vi "Actor Core.vi"(8 "error in":errorcluster, 11 "Measure Object in":refnum<class "TDMS Properties.lvclass">) -> (0 "error out":errorcluster, 3 "Actor out":refnum<class "Actor.lvclass">)   [LabVIEW 2019, in "TDMS Properties.lvclass"]
doc: "(<B>Filename</B>: Actor Framework.lvlib:Actor.lvclass:Actor Core.vi)\n\nReceives messages to the actor, reacts to them, and initiates any error handling that may shut the actor down.\n\nDescendant classes may override this VI to append parallel tasks for the actor to complete while it handles messages. Overrides use the Call Parent Method node."
uses:
  TDMS Properties.lvclass
  C:/GitHub/LabActor/Template Module/Template Module.lvclass
  C:/Program Files/National Instruments/LabVIEW 2019/vi.lib/ActorFramework/Actor/Actor.lvclass
  <vilib>/ActorFramework/Actor/Actor.lvclass
  <vilib>/Utility/tdmsutil.llb/fileViewerConfigData.ctl
  TDMS Properties.lvclass/TDMS Properties.ctl
  Template Module/Template Module.lvclass/Template Module.ctl
  <vilib>/ActorFramework/Actor/Actor.lvclass/Actor.ctl
  <vilib>/ActorFramework/Message Enqueuer/Message Enqueuer.lvclass/Message Enqueuer.ctl
  <vilib>/Utility/error.llb/DialogType.ctl
  Read File.vi
  Template Module/Read stop event.vi
  <vilib>/ActorFramework/Message Enqueuer/Init from Existing Queue.vi
  <vilib>/ActorFramework/Message Enqueuer/Enqueue.vi
  <vilib>/ActorFramework/Stop Msg/Stop Msg.lvclass
  C:/Program Files/National Instruments/LabVIEW 2019/vi.lib/ActorFramework/Message/Message.lvclass
  <vilib>/ActorFramework/Message Priority Queue/Priority Enqueue.vi
  Template Module/Template Module.lvclass
  <vilib>/ActorFramework/Message Enqueuer/Message Enqueuer.lvclass
panel:
  in  "Quit":bool
  in  "Properties":i32(listbox)
  out "file path out":path
  in  "File contents":string(tree)
  in  "Settings...":bool
  in  "Status":string
  in  "Help":bool
  in  "LastTopLeftValue":u64
  out "Temp Configuration":T1
  out "TotalCount":u64
  out "LastXScaleFormat":u8
  in  "Properties / Values / Graph":T2(tab)
  in  "Go To":bool
  in  "Scrollbar":u64(c297)
  in  "Raw data values":i32(listbox)
  out "Waveform Graph":waveform(dbl)[](graph)
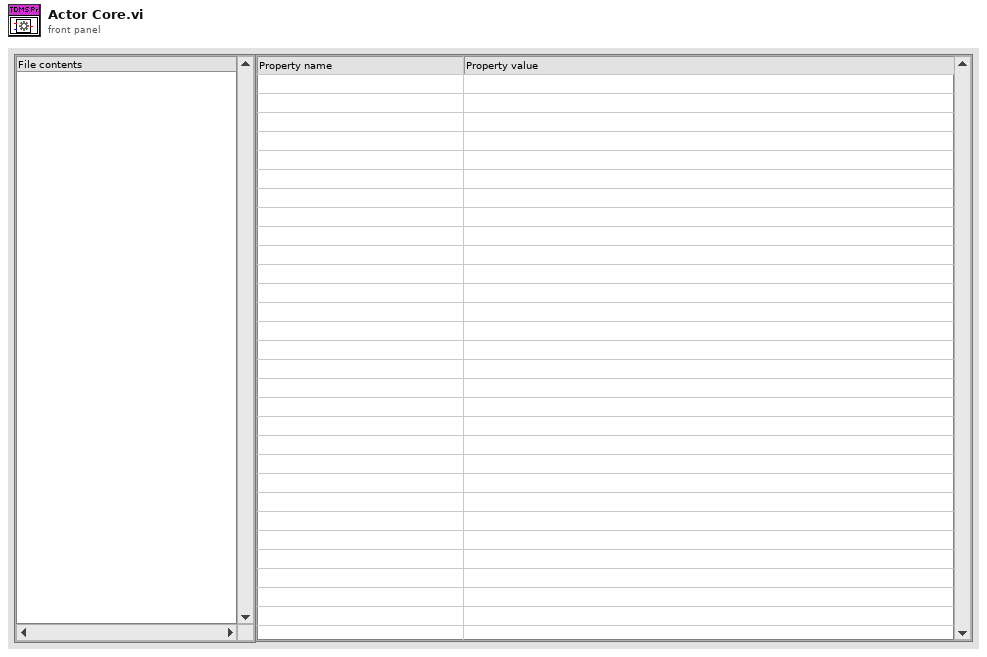
[diagram p1: front panel]
types:
  T1 = typedef "fileViewerConfigData.ctl" = cluster{"Show all (table)":bool, "Show all (graph)":bool, "limit (table)":u64, "limit (graph)":u64, "no show":bool, "start (table)":u64, "start (graph)":u64}
  T2 = enum32{"Properties", "Values (table)", "Analog values (graph)"}
  T3 = enum16{"open", "open or create", "create or replace", "create", "open (read-only)"}
  T4 = cluster{"Tree":refnum<vi>, "Tab Control":refnum<vi>, "property list":refnum<vi>, "raw data list":refnum<vi>, "Waveform Graph":refnum<vi>, "Ok":refnum<vi>, "Ok 2":refnum<vi>, "Ok 3":refnum<vi>, "Ok 4":refnum<vi>, "Scrollbar":refnum<vi>, "Ok 5":refnum<vi>, "TopLeftValue":refnum<vi>, "TotalCount":refnum<vi>}
  T5 = typedef "DialogType.ctl" = u16
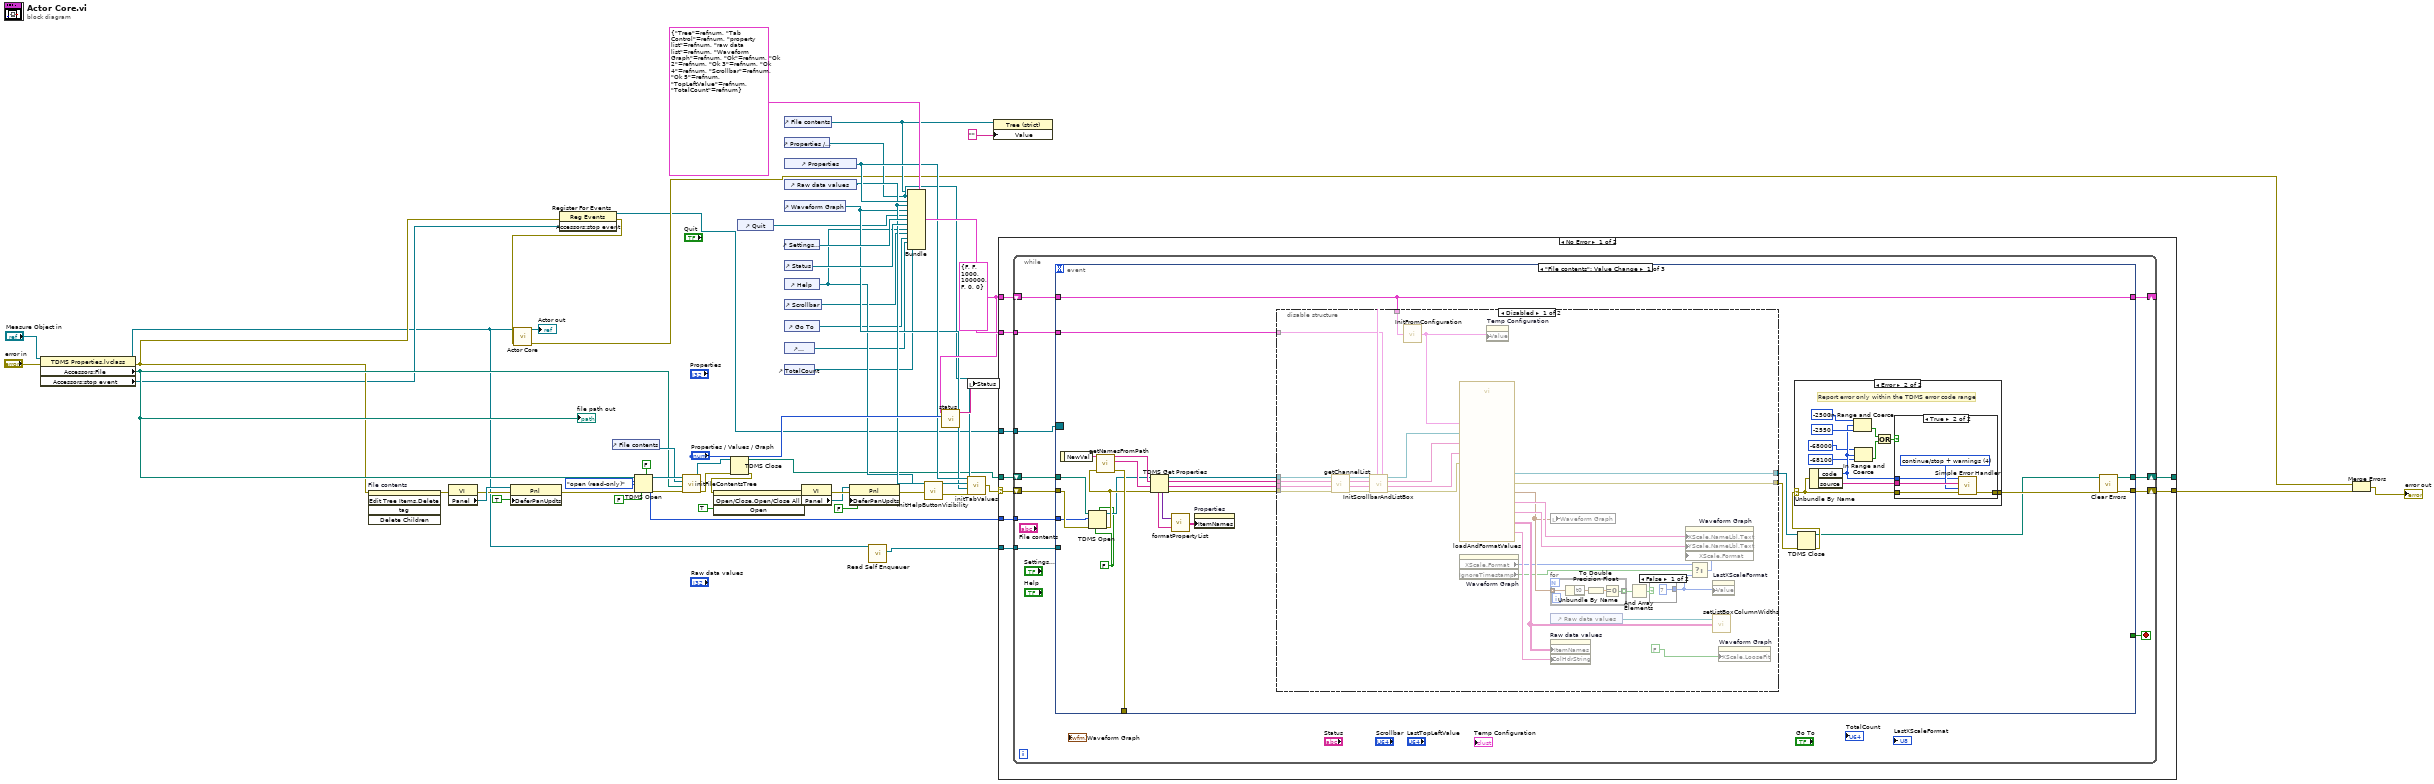
[diagram p0: block diagram]
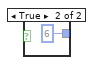
[diagram p2: hidden frame]
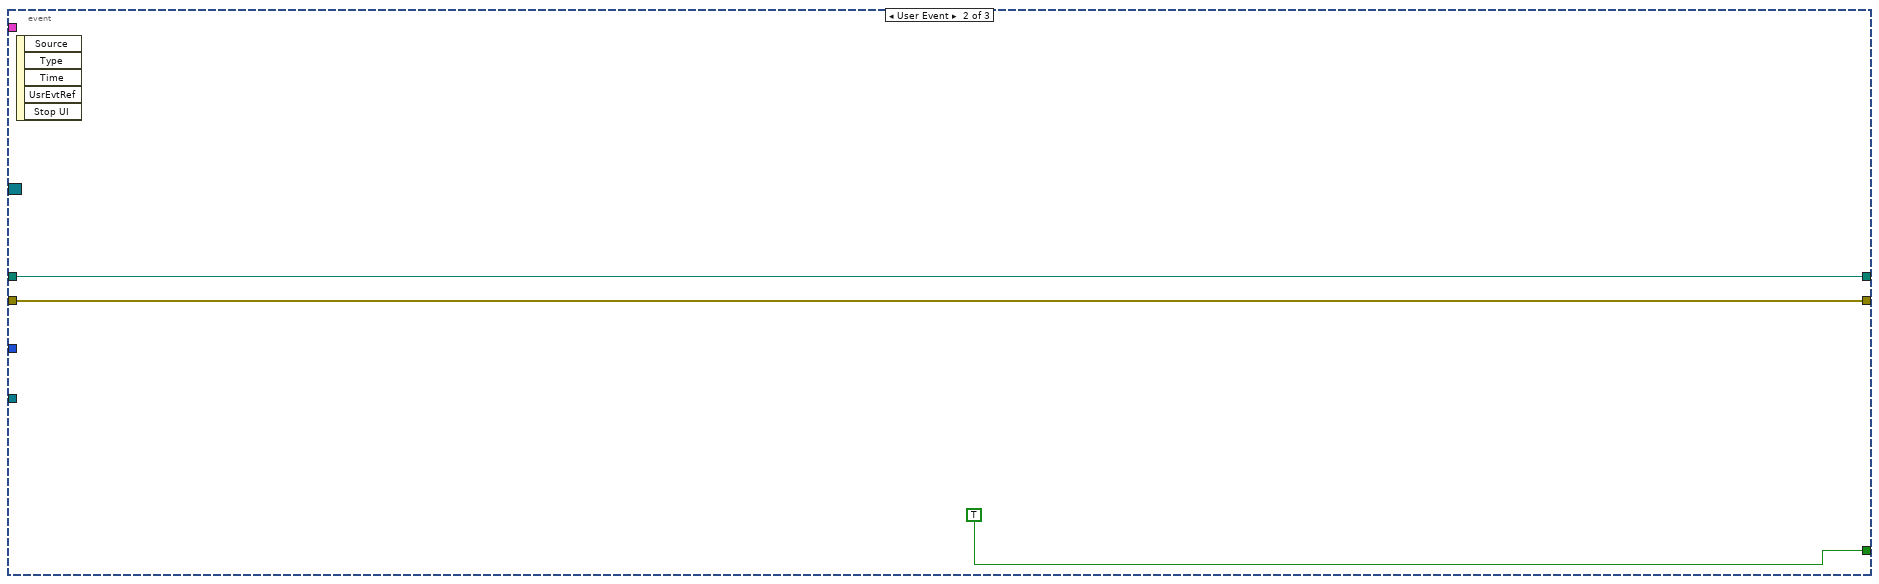
[diagram p6: hidden frame]
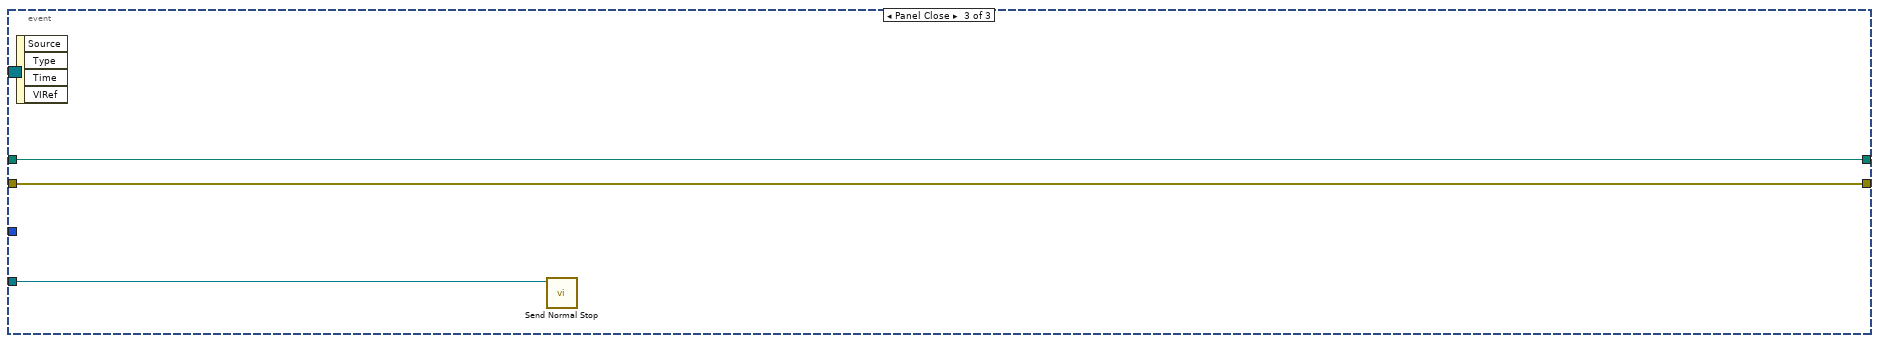
[diagram p7: hidden frame]
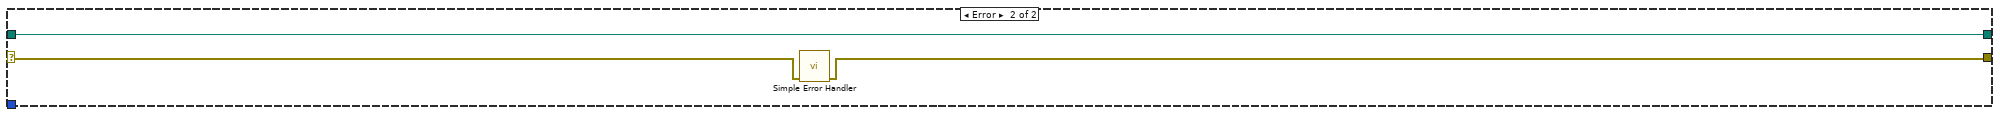
[diagram p8: hidden frame]
diagram:
  w1 = T3."open (read-only)" ("operation")
  w35 = T1 {"Show all (table)"=FALSE, "Show all (graph)"=FALSE, "limit (table)"=1000, "limit (graph)"=100000, "no show"=FALSE, "start (table)"=0, "start (graph)"=0} ("TDMS File Viewer Configuration")
  n1 = property class="TDMS Properties.lvclass"(reference="Measure Object in", error in="error in") -> (reference out=w7:refnum<class "TDMS Properties.lvclass">, error out=w11:errorcluster, "Accessors:File"=w15:path, "Accessors:stop event"=w9:refnum<user-event>)
  "file path out" <- w15
  n2 = invoke on="File contents" class="Tree (strict)" method="Edit Tree Items.Delete"(error in=w11) -> (error out=w47:errorcluster)  [unwired: 4 in, 4 out]
  n3 = property class="VI"(error in=w47) -> (error out=w48:errorcluster, "Panel"=w49:refnum<vi>)  [unwired: 1 in, 1 out]
  n4 = property class="Pnl"(reference=w49, error in=w48, "DeferPanUpdts"=TRUE ("Defer Panel Updates")) -> (error out=w51:errorcluster)  [unwired: 1 out]
  n5 = register-events(error in=w11, w9) -> (reference out=w8:refnum<event-registration>, error out=w10:errorcluster)  [unwired: 1 in]
  n6 = call-parent "Actor Core.vi"("error in"=w10, "Measure Object in"=w7) -> ("error out"=w12:errorcluster, "Actor out"=→"Actor out":refnum<class "Actor.lvclass">)  [unwired: 8 in]
  n7 = control-ref of="File contents"() -> (w38:refnum<vi>)
  n8 = TDMS Open(5:FALSE ("create index file? (T)"), 6:FALSE ("disable buffering (T)"), 8:w51, 10:w1, 11:w15) -> (0:w53:errorcluster, 3:w52:refnum<k34>)  [unwired: 2 in]
  n9 = call <vilib>:"initFileContentsTree.vi"("error in (no error)"=w53, "file path"=w15, "Tree Refnum"=w38, "tdms file"=w52) -> ("error out"=w5:errorcluster, "tdms file out"=w3:refnum<k34>)  [unwired: 2 out]
  n10 = TDMS Close(8:w5, 11:w3) -> (0:w4:errorcluster, 3:w2:path)
  n11 = invoke on="File contents" class="Tree (strict)" method="Open/Close.Open/Close All"(error in=w4, "Open"=TRUE ("Open?")) -> (error out=w43:errorcluster)  [unwired: 2 in, 3 out]
  n12 = control-ref of="Quit"() -> (w14:refnum<vi>)
  n13 = control-ref of="File contents"() -> (w26:refnum<vi>)
  n14 = control-ref of="Properties"() -> (w30:refnum<vi>)
  n15 = control-ref of="Raw data values"() -> (w29:refnum<vi>)
  n16 = control-ref of="Waveform Graph"() -> (w28:refnum<vi>)
  n17 = control-ref of="Settings..."() -> (w39:refnum<vi>)
  n18 = control-ref of="Status"() -> (w37:refnum<vi>)
  n19 = control-ref of="Help"() -> (w22:refnum<vi>)
  n20 = control-ref of="Scrollbar"() -> (w21:refnum<vi>)
  n21 = control-ref of="Go To"() -> (w20:refnum<vi>)
  n22 = control-ref of="LastTopLeftValue"() -> (w19:refnum<vi>)
  n23 = control-ref of="TotalCount"() -> (w18:refnum<vi>)
  n24 = control-ref of="Properties / Values / Graph"() -> (w27:refnum<vi>)
  n25 = property class="VI"(error in=w43) -> (error out=w45:errorcluster, "Panel"=w44:refnum<vi>)  [unwired: 1 in, 1 out]
  n26 = property class="Pnl"(reference=w44, error in=w45, "DeferPanUpdts"=FALSE ("Defer Panel Updates")) -> (error out=w24:errorcluster)  [unwired: 1 out]
  n27 = call <vilib>:"Read Self Enqueuer.vi"("Actor"=w7) -> ("Self Enqueuer"=w6:refnum<class "Message Enqueuer.lvclass">)  [unwired: 10 in]
  n28 = Bundle(cluster=T4 {"Tree"=refnum, "Tab Control"=refnum, "property list"=refnum, "raw data list"=refnum, "Waveform Graph"=refnum, "Ok"=refnum, "Ok 2"=refnum, "Ok 3"=refnum, "Ok 4"=refnum, "Scrollbar"=refnum, "Ok 5"=refnum, "TopLeftValue"=refnum, "TotalCount"=refnum} ("control refs"), "Tree"=w26, "Tab Control"=w27, "property list"=w30, "raw data list"=w29, "Waveform Graph"=w28, "Ok"=w14, "Ok 2"=w39, "Ok 3"=w37, "Ok 4"=w22, "Scrollbar"=w21, "Ok 5"=w20, "TopLeftValue"=w19, "TotalCount"=w18) -> (w41:T4)
  n29 = call <vilib>:"initHelpButtonVisibility.vi"("error in"=w24, "Help"=w22) -> ("error out"=w23:errorcluster)  [unwired: 9 in]
  n30 = call <vilib>:"status.vi"("tab sheet"="Properties / Values / Graph", "TDMS File Viewer Configuration"=w35) -> ("status"=w36:string)  [unwired: 5 out]
  n31 = local write "Status"(w36) -> ()
  n32 = call <vilib>:"initTabValues.vi"("properties"=w30, "Values"=w29, "waveform"=w28, "error in"=w23, "Properties / Values / Graph"=w27) -> ("error out"=w31:errorcluster)
  n33 = property class="Tree (strict)"(reference=w26, "Value"="") -> ()  [unwired: 1 in, 2 out]
  n34 = case shown="No Error" w31 {
    selector: w31 -> [w59 w164]
    tunnel: w2 -> [w64 w165]
    tunnel: [w63 w165] -> _
    tunnel: [w62 w163] -> w33
    tunnel: w41 -> [w61 _]
    tunnel: w35 -> [w60 _]
    tunnel: w8 -> [w58 _]
    tunnel: w6 -> [w57 _]
    tunnel: w1 -> [w56 _]
    frame No Error {
      n35 = while {
        shift-right: [w73] -> w62
        shift-left: w59 -> [w74]
        shift-right: [w72] -> w63
        shift-left: w64 -> [w75]
        tunnel: w61 -> [w71]
        shift-right: [w69] -> _
        shift-left: w60 -> [w70]
        tunnel: w58 -> [w68]
        tunnel: w57 -> [w66]
        tunnel: w56 -> [w65]
        stop <- w67 stop-if-true
        n36 = event shown="[0] \"File contents\": Value Change" {
          selector: w68 -> [_ _ _]
          dyn-events: _ -> [_ _ _]
          timeout: _ -> [_ _ _]
          tunnel: w75 -> [w83 w158 w161]
          tunnel: w74 -> [w85 w157 w160]
          tunnel: [w93 w157 w160] -> w73
          tunnel: [w78 w158 w161] -> w72
          tunnel: [w94 _ _] -> _
          tunnel: w71 -> [w86 _ _]
          tunnel: w70 -> [w87 _ _]
          tunnel: [w87 _ _] -> w69
          tunnel: [_ TRUE _] -> w67
          tunnel: w66 -> [_ _ w162]
          tunnel: w65 -> [w76 _ _]
          event "File contents": Value Change {
            w77 = FALSE ("create index file? (T)")
            n37 = event-data() -> ("NewVal"=w96:string)  [unwired: 1 out]
            n38 = TDMS Open(5:w77, 6:w77, 8:w85, 10:w76, 11:w83) -> (0:w84:errorcluster, 3:w82:refnum<k34>)  [unwired: 2 in]
            n39 = call <vilib>:"getNamesFromPath.vi"("error in (no error)"=w84, "tree path"=w96) -> ("error out"=w94:errorcluster, "channel"=w99:string, "group"=w100:string)  [unwired: 3 out]
            n40 = TDMS Get Properties(8:w84, 9:w99, 10:w100, 11:w82) -> (0:w91:errorcluster, 1:w90:string, 2:w89:string, 3:w92:refnum<k34>, 4:w97:variant[], 6:w98:string[])  [unwired: 2 out]
            n41 = call <vilib>:"formatPropertyList.vi"("property names"=w98, "property values"=w97) -> ("strings"=w95:string[][])
            n42 = property on="Properties" class="MCListbox (strict)"("ItemNames"=w95) -> ()  [unwired: 2 in, 2 out]
            n43 = disable-structure shown="Disabled" {
              disable-tunnel: [w130 w137] -> w79
              disable-tunnel: w92 -> [w127 w137]
              disable-tunnel: w91 -> [w126 w138]
              disable-tunnel: w90 -> [w125 _]
              disable-tunnel: w89 -> [w121 _]
              disable-tunnel: [w120 w138] -> w81
              disable-tunnel: w87 -> [w109 _]
              disable-tunnel: w86 -> [w108 _]
              frame Disabled {
                n44 = call <vilib>:"getChannelList.vi"("error in (no error)"=w126, "channel names"=w125, "group name"=w121, "tdms file"=w127) -> ("error out"=w117:errorcluster, "channel names out"=w115:string[], "group names out"=w113:string[], "tdms file out"=w111:refnum<k34>)
                n45 = call <vilib>:"InitScrollbarAndListBox.vi"("control refs"=w108, "configuration"=w109, "error in (no error)"=w117, "channel names"=w115, "group names"=w113, "tdms in"=w111) -> ("error out"=w116:errorcluster, "channel out"=w114:string[], "group out"=w112:string[], "tdms out"=w110:refnum<k34>)  [unwired: 2 in]
                n46 = call <vilib>:"InitFromConfiguration.vi"("configuration"=w109) -> ("output cluster"=w118:T1)  [unwired: 4 in]
                n47 = call <vilib>:"loadAndFormatValues.vi"("error in (no error)"=w116, "configuration"=w118, "channel names"=w114, "group names"=w112, "tdms file"=w110) -> ("error out"=w120:errorcluster, "graph y names"=w123:string, "graph x names"=w122:string, "tdms file out"=w130:refnum<k34>, "waveform values"=w107:waveform(dbl)[], "table values"=w129:string[][], "table headers"=w124:string[])
                n48 = property on="Waveform Graph" class="WFGraph (strict)"() -> ("XScale.Format"=w102:u8, "IgnoreTimestamp"=w101:bool)  [unwired: 2 in, 2 out]
                n49 = property on="Temp Configuration" class="Clust (strict)"("Value"=w118) -> ()  [unwired: 2 in, 2 out]
                n50 = local write "Waveform Graph"(w107) -> ()
                n51 = for {
                  tunnel: w107 -> [w136] mode=indexing
                  tunnel: [w133] -> w106 mode=indexing
                  n52 = Unbundle By Name(w136) -> ("t0"=w135:timestamp)
                  n53 = To Double Precision Float(number=w135) -> (double precision float=w134:dbl)
                  n54 = Equal To 0?(x=w134) -> (x = 0?=w133:bool)
                }
                n55 = control-ref of="Raw data values"() -> (w128:refnum<vi>)
                n56 = property on="Raw data values" class="MCListbox (strict)"("ItemNames"=w129, "ColHdrString"=w124) -> ()  [unwired: 2 in, 2 out]
                n57 = And Array Elements(Boolean array=w106) -> (logical AND=w105:bool)
                n58 = case shown="False" w105 {
                  tunnel: [u8 7 u8 6] -> w103
                  frame False {
                  }
                  frame True {
                  }
                }
                n59 = Select(t=w102, s=w101, f=w103) -> (s? t:f=w104:u8)
                n60 = property on="Waveform Graph" class="WFGraph (strict)"("XScale.NameLbl.Text"=w122, "YScale.NameLbl.Text"=w123, "XScale.Format"=w104) -> ()  [unwired: 2 in, 2 out]
                n61 = property on="LastXScaleFormat" class="DigNum (strict)"("Value"=w103) -> ()  [unwired: 2 in, 2 out]
                n62 = call <vilib>:"setListBoxColumnWidths.vi"("table data"=w129, "MCListbox Refnum"=w128) -> ()  [unwired: 1 out]
                n63 = property on="Waveform Graph" class="WFGraph (strict)"("XScale.LooseFit"=FALSE ("X Scale.Loose Fit")) -> ()  [unwired: 2 in, 2 out]
              }
              frame Enabled {
              }
            }
            n64 = TDMS Close(8:w81, 11:w79) -> (0:w80:errorcluster, 3:w78:path)
            n65 = case shown="Error" w80 {
              selector: w80 -> [w139 w149]
              tunnel: [w139 w148] -> w88
              frame No Error {
              }
              frame Error {
                # "Report error only within the TDMS error code range"
                n66 = Unbundle By Name(w149) -> ("code"=w145:i32, "source"=w150:string)
                n67 = In Range and Coerce(upper limit=-2500, x=w145, lower limit=-2550 ("upper limit")) -> (In Range?=w142:bool)  [unwired: 1 out]
                n68 = In Range and Coerce(upper limit=-68000, x=w145, lower limit=-68100) -> (In Range?=w141:bool)  [unwired: 1 out]
                n69 = Or(x=w142, y=w141) -> (x .or. y?=w140:bool)
                n70 = case shown="True" w140 {
                  tunnel: w150 -> [_ w156]
                  tunnel: w149 -> [w151 w155]
                  tunnel: [w151 w154] -> w148
                  tunnel: w145 -> [_ w152]
                  frame False {
                    # "Out of the range of TDMS\nerror code, we don't report\nthem."
                  }
                  frame True {
                    w153 = T5 4 items=["no dialog", "OK message", "continue or stop message", "OK message + warnings", "continue/stop + warnings"] ("type of dialog (OK msg:1)")
                    n71 = call <vilib>:"Simple Error Handler.vi"("error code (no error:0)"=w152, "error source (\" \")"=w156, "type of dialog (OK msg:1)"=w153, "error in (no error)"=w155) -> ("error out"=w154:errorcluster)  [unwired: 1 in, 4 out]
                  }
                }
              }
            }
            n72 = call <vilib>:"Clear Errors.vi"("error in (no error)"=w88) -> ("error out"=w93:errorcluster)  [unwired: 1 in, 5 out]
          }
          event User Event {
            n73 = event-data() -> ()  [unwired: 6 out]
          }
          event Panel Close {
            n74 = event-data() -> ()  [unwired: 5 out]
            n75 = call <vilib>:"Send Normal Stop.vi"("Message Enqueuer"=w162) -> ()  [unwired: 10 in, 1 out]
          }
        }
      }
    }
    frame Error {
      n76 = call <vilib>:"Simple Error Handler.vi"("error in (no error)"=w164) -> ("error out"=w163:errorcluster)  [unwired: 1 in, 7 out]
    }
  }
  n77 = Merge Errors(w12, w33) -> (→"error out":errorcluster)
